vi "Humidity.vi"(8 "error in (no error)":errorcluster) -> (0 "error out":errorcluster, 2 "Cashew Humidity":dbl(knob) scale=0.0..120.0)   [LabVIEW 2018]
uses:
  <vilib>/express/express arith-compare/Formula/XNode/ExpressFormulaBlockNode.xnode
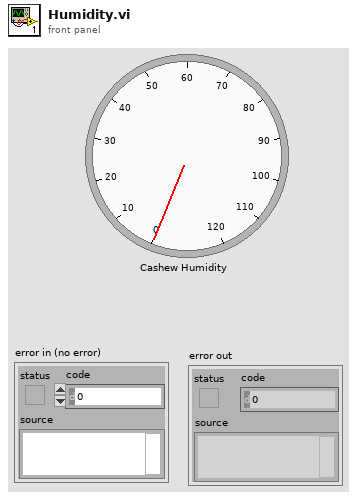
[diagram p1: front panel]
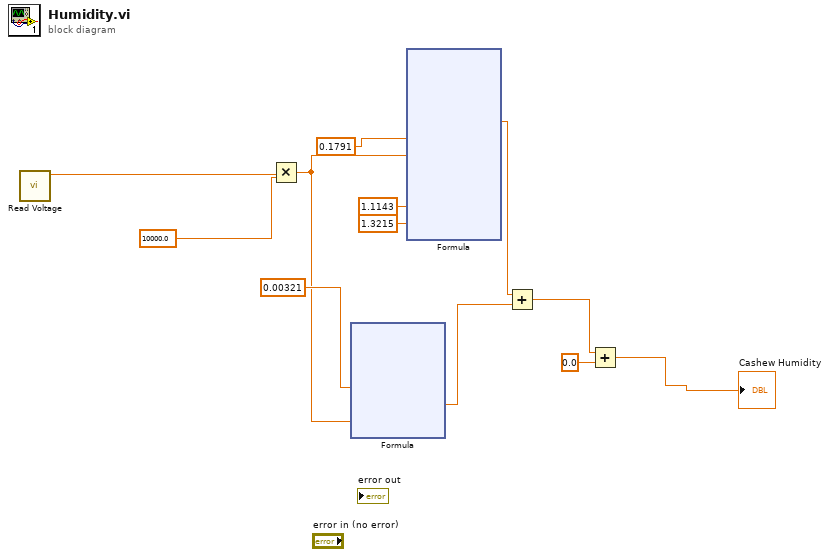
[diagram p0: block diagram]
diagram:
  n1 = call "Read Voltage.vi"() -> ("voltage"=w12:dbl)  [unwired: 1 in, 6 out]
  n2 = Multiply(x=w12, y=10000.0) -> (x*y=w8:dbl)
  n3 = xnode "Formula"("b"=0.00321, "t"=w8) -> ("Result"=w6:dbl)  [unwired: 1 in, 1 out]
  n4 = xnode "Formula"("K"=0.1791, "t"=w8, "a"=1.1143, "n"=1.3215) -> ("Result"=w7:dbl)  [unwired: 1 in, 1 out]
  n5 = Add(x=w7, y=w6) -> (x+y=w5:dbl)
  n6 = Add(x=w5, y=0.0) -> (x+y=→"Cashew Humidity":dbl)
